vi "MVP01.vi"() -> ()   [LabVIEW 2016]
uses:
  Controls/Teste Case Selector 01.ctl
  <vilib>/xnet/xnet.llb/XNET Write (Signal Single-point).vi
panel:
  in  "Enum":T1=enum."Caso 2,Valor 2"
  out "Gabarito":string
  out "String (OCR/OCV 1)":string
  out "Passed?":bool
  in  "Menu":dbl[](array[numeric])=[0.0]
  in  "milliseconds to wait":u32=100
  in  "stop":bool
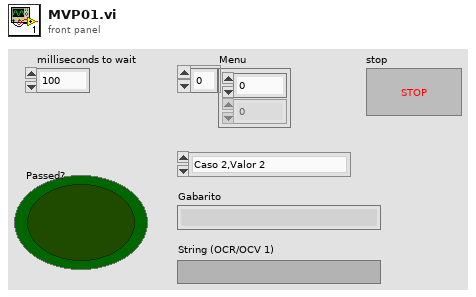
[diagram p1: front panel]
types:
  T1 = typedef "Teste Case Selector 01.ctl" = enum16{"Outros", "Caso 2,Valor 1", "Caso 2,Valor 2"}
  T2 = typedef "IMAQ Image.ctl" = refnum<image>
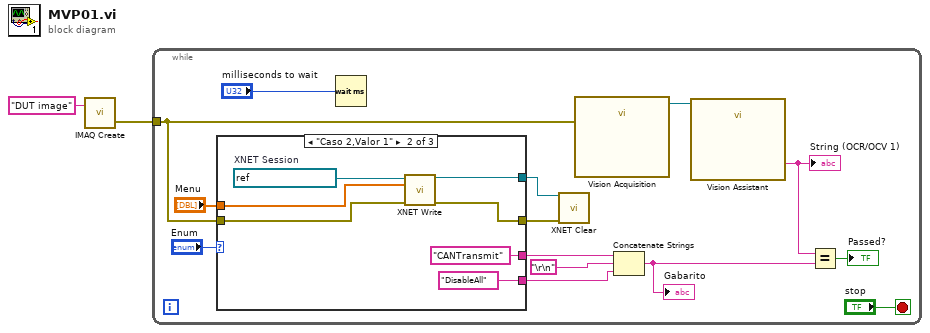
[diagram p0: block diagram]
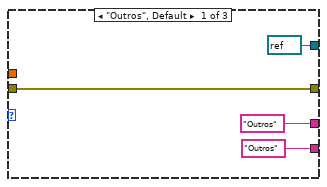
[diagram p2: hidden frame]
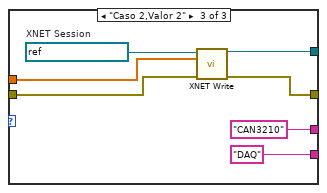
[diagram p3: hidden frame]
diagram:
  n1 = call "IMAQ Create"("Image Name"="DUT image") -> ("error out"=w1:errorcluster)  [unwired: 4 in, 1 out]
  n2 = while {
    tunnel: w1 -> [w5]
    stop <- "stop" stop-if-true
    n3 = case shown="\"Caso 2,Valor 1\"" "Enum" {
      tunnel: ["Outros" "CANTransmit" "CAN3210"] -> w10
      tunnel: ["Outros" "DisableAll" "DAQ"] -> w8
      tunnel: [w18 w25 w32] -> w7
      tunnel: [refnum<k21> refnum ("session out") w24 w31] -> w6
      tunnel: w5 -> [w18 w23 w30]
      tunnel: "Menu" -> [_ w21 w28]
      frame "Outros", Default {
      }
      frame "Caso 2,Valor 1" {
        w22 = refnum<k21> "Set LCD Menu"  # XNET Session
        n4 = call-poly <vilib>:"XNET Write.vi"("session in"=w22, "data"=w21, "error in (no error)"=w23) -> ("session out"=w24:refnum<k21>, "error out"=w25:errorcluster)  [unwired: 11 in]
      }
      frame "Caso 2,Valor 2" {
        w29 = refnum<k21> "Set LCD Menu"  # XNET Session
        n5 = call-poly <vilib>:"XNET Write.vi"("session in"=w29, "data"=w28, "error in (no error)"=w30) -> ("session out"=w31:refnum<k21>, "error out"=w32:errorcluster)  [unwired: 11 in]
      }
    }
    n6 = Wait (ms)(milliseconds to wait="milliseconds to wait") -> ()  [unwired: 1 out]
    n7 = call <vilib>:"XNET Clear.vi"("session in"=w6, "error in (no error)"=w7) -> ()  [unwired: 13 in, 1 out]
    n8 = call "Vision Acquisition"("error in"=w5) -> ("Image Out"=w12:T2)  [unwired: 25 in, 1 out]
    n9 = Concatenate Strings(w10, "\r\n", w8) -> (w11:string)
    "Gabarito" <- w11
    n10 = call "Vision Assistant"("Image In"=w12) -> ("String (OCR/OCV 1)"=w14:string)  [unwired: 24 in, 2 out]
    "String (OCR/OCV 1)" <- w14
    n11 = Equal?(x=w14, y=w11) -> (x = y?=→"Passed?":bool)
  }
